vi "MultipleChannelEditorUI.vi"(8 "error in":errorcluster, 11 "SequenceRepo in":refnum<class "SequenceRepo.lvclass">) -> (0 "error out":errorcluster, 3 "SequenceRepo out":refnum<class "SequenceRepo.lvclass">)   [LabVIEW 2015, in "SequenceRepo.lvclass"]
doc: "Copyright 2017 National Instruments Corporation\n\nLicensed under the Apache License, Version 2.0 (the \"License\"); you may not use this file except in compliance with the License. You may obtain a copy of the License at http://www.apache.org/licenses/LICENSE-2.0\nUnless required by applicable law or agreed to in writing, software distributed under the License is distributed on an \"AS IS\" BASIS, WITHOUT WARRANTIES OR CONDITIONS OF ANY KIND, either express or implied. See the License for the specific language governing permissions and limitations under the License."
uses:
  SequenceRepo.lvclass
panel:
  in  "Table":string[][](table)
  in  "Cancel":bool
  in  "OK":bool
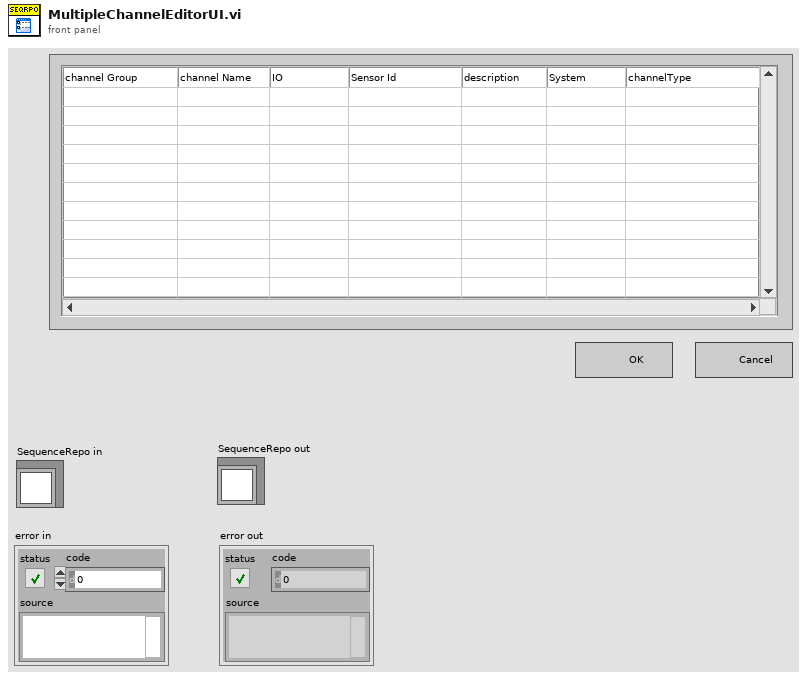
[diagram p1: front panel]
types:
  T1 = enum32{"Invalid", "Standard", "Closed", "Hidden", "Minimized", "Maximized"}
  T2 = typedef "cRIORepo.lvclass/ChannelData.ctl" = cluster{"channel group":string, "channel name":string, "IO ":string, "sensor ID":string, "description":string, "system":string, "channel type":string}
  T3 = cluster{"Table[0]":string, "Table[1]":string, "Table[2]":string, "Table[3]":string, "Table[4]":string, "Table[5]":string, "Table[6]":string}
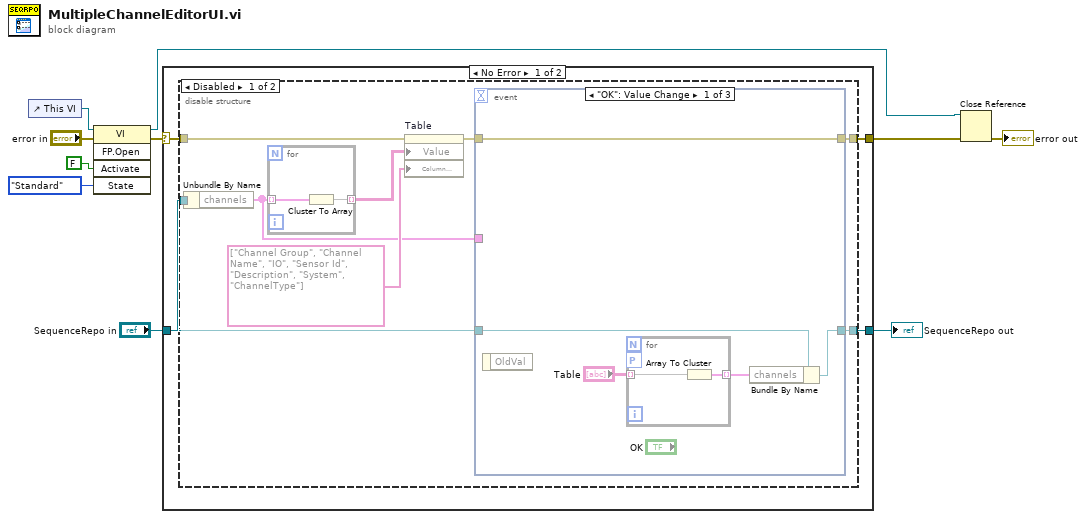
[diagram p0: block diagram]
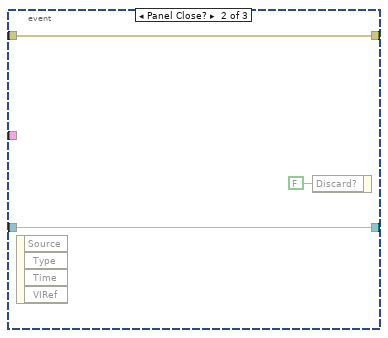
[diagram p2: hidden frame]
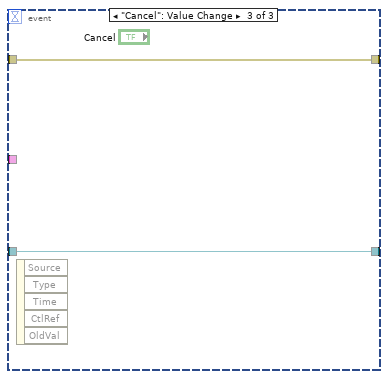
[diagram p3: hidden frame]
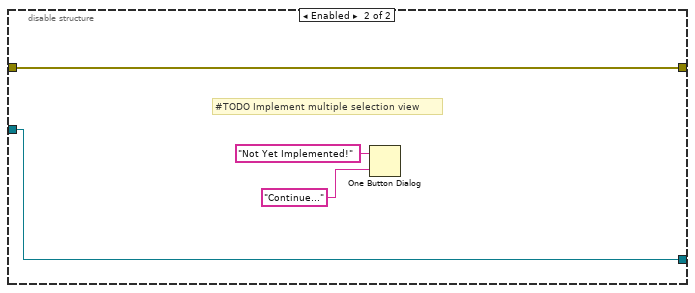
[diagram p4: hidden frame]
diagram:
  n1 = control-ref of="This VI"() -> (w7:refnum<vi>)
  n2 = invoke class="VI" method="FP.Open"(reference=w7, error in="error in", "Activate"=FALSE ("Activate?"), "State"=T1."Standard") -> (reference out=w2:refnum<vi>, error out=w3:errorcluster)  [unwired: 1 in, 3 out]
  n3 = case shown="No Error" w3 {
    selector: w3 -> [w14 w42]
    tunnel: "SequenceRepo in" -> [w12 w41]
    tunnel: [w11 w41] -> w9
    tunnel: [w13 w42] -> w1
    frame No Error {
      n4 = disable-structure shown="Disabled" {
        disable-tunnel: w14 -> [w22 w40]
        disable-tunnel: [w21 w40] -> w13
        disable-tunnel: w12 -> [w16 w39]
        disable-tunnel: [w15 w39] -> w11
        frame Disabled {
          n5 = Unbundle By Name(w16) -> ("channels"=w17:T2[])
          n6 = for {
            tunnel: w17 -> [w24] mode=indexing
            tunnel: [w23] -> w20 mode=indexing
            n7 = Cluster To Array(cluster=w24) -> (array=w23:string[])
          }
          n8 = property on="Table" class="Tbl (strict)"(error in=w22, "Value"=w20, "Column Headers[]"=string[] ["Channel Group", "Channel Name", "IO", "Sensor Id", "Description", "System", "ChannelType"] ("Column Header Strings[]")) -> (error out=w19:errorcluster)  [unwired: 1 in, 1 out]
          n9 = event shown="[0] \"OK\": Value Change" {
            selector: _ -> [_ _ _]
            dyn-events: _ -> [_ _ _]
            timeout: _ -> [_ _ _]
            tunnel: w19 -> [w29 w33 w35]
            tunnel: [w29 w33 w35] -> w21
            tunnel: w17 -> [_ _ _]
            tunnel: w16 -> [w27 w32 w36]
            tunnel: [w26 w32 w36] -> w15
            event "OK": Value Change {
              n10 = event-data() -> ()  [unwired: 1 in, 1 out]
              n11 = for {
                tunnel: "Table" -> [w31] mode=indexing
                tunnel: [w30] -> w25 mode=indexing
                workers-P: _ -> [_]
                n12 = Array To Cluster(array=w31) -> (cluster=w30:T3)
              }
              n13 = Bundle By Name(cluster=w27, "channels"=w25) -> (w26:refnum<class "SequenceRepo.lvclass">)
            }
            event Panel Close? {
              n14 = event-data() -> ()  [unwired: 1 in, 4 out]
              n15 = event-data("Discard?"=FALSE) -> ()  [unwired: 1 in, 1 out]
            }
            event "Cancel": Value Change {
              n16 = event-data() -> ()  [unwired: 1 in, 5 out]
            }
          }
        }
        frame Enabled {
          # "#TODO Implement multiple selection view"
          n17 = One Button Dialog(message="Not Yet Implemented!", button name ("OK")="Continue...") -> ()  [unwired: 1 out]
        }
      }
    }
    frame Error {
    }
  }
  "SequenceRepo out" <- w9
  n18 = Close Reference(reference=w2, error in (no error)=w1) -> (error out=→"error out":errorcluster)
